vi "Axis Send Cmd.vi"(10 "DataIn":cluster{"Action":string, "Data":variant}={"Action"="Check Home", "Data"=variant}, 11 "Axis Index":i32=2) -> (0 "Error Out":errorcluster)   [LabVIEW 2019]
uses:
  LLB/Commonly VI.lvlib
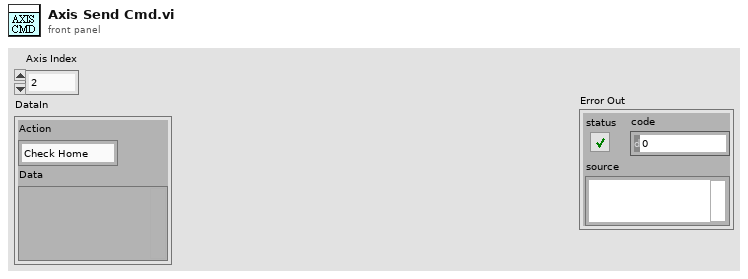
[diagram p1: front panel]
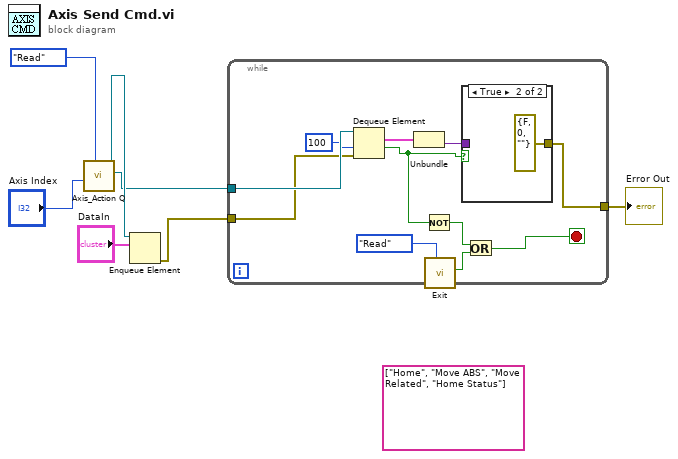
[diagram p0: block diagram]
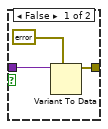
[diagram p2: hidden frame]
diagram:
  (unwired) string[] ["Home", "Move ABS", "Move Related", "Home Status"]
  n1 = call "Axis_Action Q.vi"("Enum"=enum16{"Initial", "Write", "Read"}."Read", "Axis Index"="Axis Index") -> ("Axis ActFeedBackQ Out"=w5:refnum<queue>, "Axis ActQ Out"=w6:refnum<queue>)  [unwired: 7 in, 1 out]
  n2 = Enqueue Element(queue=w6, element="DataIn") -> (error out=w4:errorcluster)  [unwired: 2 in, 2 out]
  n3 = while {
    tunnel: w5 -> [w18]
    tunnel: w4 -> [w17]
    tunnel: [w13] -> w1
    stop <- w9 stop-if-true
    n4 = Dequeue Element(queue=w18, timeout in ms (-1)=100, error in (no error)=w17) -> (element=w15:cluster{"Action":string, "Data":variant}, timed out?=w8:bool)  [unwired: 2 out]
    n5 = Unbundle(w15) -> ("Data"=w14:variant)  [unwired: 1 out]
    n6 = Not(x=w8) -> (.not. x?=w12:bool)
    n7 = call "Exit.vi"("Enum"=enum16{"Initial", "Read", "Write"}."Read") -> ("ExitOut"=w11:bool)  [unwired: 10 in]
    n8 = case shown="True" w8 {
      tunnel: w14 -> [w21 _]
      tunnel: [w19 errorcluster {"status"=FALSE, "code"=0, "source"=""} ("error constant")] -> w13
      frame False {
        n9 = Variant To Data(type=errorcluster {"status"=FALSE, "code"=0, "source"=""} ("error constant"), Variant=w21) -> (data=w19:errorcluster)  [unwired: 1 in, 1 out]
      }
      frame True {
      }
    }
    n10 = Or(x=w12, y=w11) -> (x .or. y?=w9:bool)
  }
  "Error Out" <- w1
